vi "ConvertStrings(Hex to Normal).vi"(11 "Hex String":string="H\f\u0000D\u0014\u0014") -> (3 "Normal String":string)   [LabVIEW 2010]
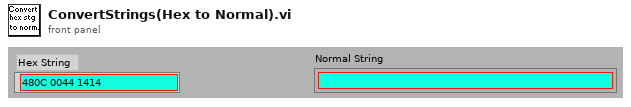
[diagram p1: front panel]
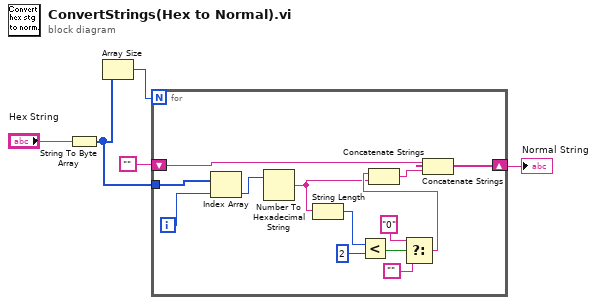
[diagram p0: block diagram]
diagram:
  n1 = String To Byte Array(string="Hex String") -> (unsigned byte array=w4:u8[])
  n2 = Array Size(array=w4) -> (size(s)=w5:i32)
  n3 = for {
    N: w5 -> [_]
    shift-right: [w15] -> w2
    shift-left: "" -> [w8]
    tunnel: w4 -> [w17]
    i -> [w18]
    n4 = Index Array(array=w17, index=w18) -> (element=w16:u8)
    n5 = Number To Hexadecimal String(2:w16) -> (0:w7:string)  [unwired: 1 out]
    n6 = String Length(string=w7) -> (length=w14:i32)
    n7 = Less?(x=w14, y=2) -> (x < y?=w12:bool)
    n8 = Select(t="0", s=w12, f="") -> (s? t:f=w9:string)
    n9 = Concatenate Strings(w9, w7) -> (w6:string)
    n10 = Concatenate Strings(w8, w6) -> (w15:string)
  }
  "Normal String" <- w2
